vi "PrepareAcquisitionSD.vi"(2 "error in (no error)":errorcluster) -> (0 "error out":errorcluster, 1 "DLL error code":u32)   [LabVIEW 2015]
doc: "The <B>PrepareAcquisition</B> function reads the current acquisition setup and allocates and clears any memory that will be used during the acquisition. The function call is not required as it will be called automatically by the <B>StartAcquisition</B> function if it has not already been called externally. However for long kinetic series acquisitions the time to allocate and clear any memory can be quite long which can result in a long delay between calling <B>StartAcquisition</B> and the acquisition actually commencing. Calling <B>PrepareAcquisition</B> first will reduce this delay in the <B>StartAcquisition</B> call.\n\n<B>Error codes:</B>\nDRV_SUCCESS - Acquisition prepared.\nDRV_NOT_INITIALIZED - System not initialized.\nDRV_ACQUIRING - Acquisition in progress.\nDRV_VXDNOTINSTALLED - VxD not loaded.\nDRV_ERROR_ACK - Unable to communicate with card.\nDRV_INIERROR - Error reading \"DETECTOR.INI\".\nDRV_ACQUISITION_ERRORS - Acquisition settings invalid.\nDRV_ERROR_PAGELOCK - Unable to allocate memory.\nDRV_INVALID_FILTER - Filter not available for current acquisition.\nDRV_IOCERROR - Integrate On Chip setup error."
uses:
  DLL/atmcd32d.dll
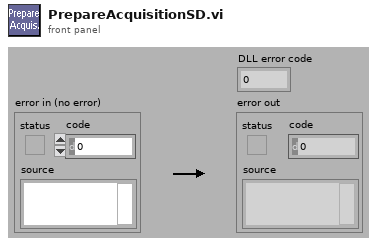
[diagram p1: front panel]
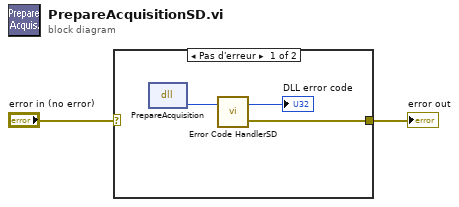
[diagram p0: block diagram]
diagram:
  n1 = case shown="Pas d'erreur" "error in (no error)" {
    selector: "error in (no error)" -> [_ w6]
    tunnel: [w4 w6] -> w1
    frame No Error {
      n2 = dll-call lib="G:/SD/TRANCON/DLL/Atmcd32d.dll" fn="PrepareAcquisition"() -> (w5:u32)  [unwired: 3 in, 2 out]
      n3 = call "Error Code HandlerSD.vi"("DLL error code"=w5) -> ("error out"=w4:errorcluster, "dup DLL error code"=→"DLL error code":u32)  [unwired: 1 in]
    }
    frame Error {
    }
  }
  "error out" <- w1
